vi "ConfigOperateMode.vi"(8 "error in (no error)":errorcluster, 11 "ClassIn":refnum<class "Keysight335XX.lvclass">) -> (0 "error out":errorcluster, 3 "ClassOut":refnum<class "Keysight335XX.lvclass">)   [LabVIEW 2014, in "FGenPlugins.lvlib" / "Keysight335XX.lvclass"]
uses:
  Keysight335XX.lvclass
  <instrlib>/Agilent 3352X Series/Agilent 3352X Series.lvlib
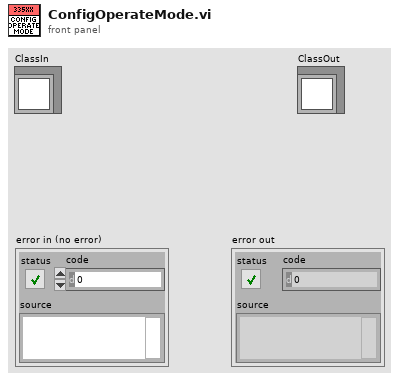
[diagram p1: front panel]
types:
  T1 = typedef "FGenPlugins.lvlib/NISTFGenPluginsBase.lvclass/ChannelParamElement.ctl" = cluster{"sName":string, "eOperateMode":u16, "bEnabled":bool, "eOutputMode":u16, "iIndex":i32, "iNameBufferSize":i32, "fGain":dbl}
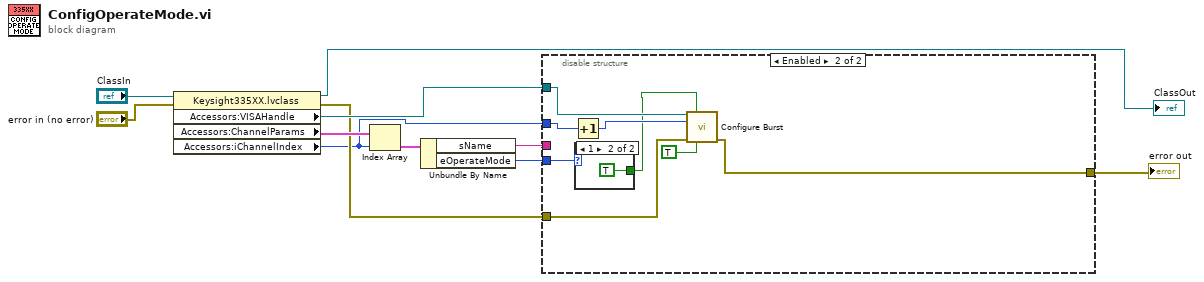
[diagram p0: block diagram]
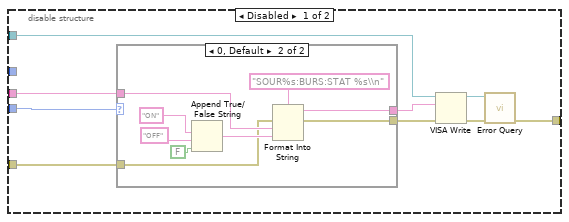
[diagram p2: hidden frame]
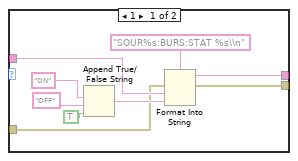
[diagram p3: hidden frame]
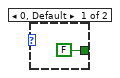
[diagram p4: hidden frame]
diagram:
  n1 = property class="Keysight335XX.lvclass"(reference="ClassIn", error in="error in (no error)") -> (reference out=→"ClassOut":refnum<class "Keysight335XX.lvclass">, error out=w6:errorcluster, "Accessors:VISAHandle"=w10:refnum<visa-resource-name>, "Accessors:ChannelParams"=w8:T1[], "Accessors:iChannelIndex"=w2:i32)
  n2 = Index Array(array=w8, index=w2) -> (element=w5:T1)
  n3 = Unbundle By Name(w5) -> ("sName"=w4:string, "eOperateMode"=w3:u16)
  n4 = disable-structure shown="Enabled" {
    disable-tunnel: w10 -> [w20 w46]
    disable-tunnel: [w19 w39] -> w9
    disable-tunnel: w6 -> [w18 w40]
    disable-tunnel: w4 -> [w13 _]
    disable-tunnel: w3 -> [w12 w43]
    disable-tunnel: w2 -> [_ w45]
    frame Disabled {
      n5 = case shown="0, Default" w12 {
        tunnel: w13 -> [w24 w33]
        tunnel: w18 -> [w23 w32]
        tunnel: [w22 w31] -> w17
        tunnel: [w21 w30] -> w16
        frame 1 {
          n6 = Append True/False String(1:TRUE ("selector"), 2:"OFF", 3:"ON") -> (0:w25:string)  [unwired: 1 out]
          n7 = Format Into String(format string="SOUR%s:BURS:STAT %s\\n", error in=w23, w24, w25) -> (resulting string=w21:string, error out=w22:errorcluster)  [unwired: 1 in]
        }
        frame 0, Default {
          n8 = Append True/False String(1:FALSE ("selector"), 2:"OFF", 3:"ON") -> (0:w34:string)  [unwired: 1 out]
          n9 = Format Into String(format string="SOUR%s:BURS:STAT %s\\n", error in=w32, w33, w34) -> (resulting string=w30:string, error out=w31:errorcluster)  [unwired: 1 in]
        }
      }
      n10 = VISA Write(VISA resource name=w20, write buffer=w16, error in (no error)=w17) -> (VISA resource name out=w15:refnum<visa-resource-name>, error out=w14:errorcluster)  [unwired: 1 out]
      n11 = call <instrlib>:"Error Query.vi"("error in (no error)"=w14, "VISA resource name"=w15) -> ("error out"=w19:errorcluster)  [unwired: 9 out]
    }
    frame Enabled {
      n12 = Increment(x=w45) -> (x+1=w44:i32)
      n13 = case shown="1" w43 {
        tunnel: [FALSE TRUE] -> w42
        frame 0, Default {
        }
        frame 1 {
        }
      }
      n14 = call <instrlib>:"Configure Burst.vi"("VISA resource name"=w46, "Enable Burst (T: Enable)"=w42, "Channel (1: 1)"=w44, "error in (no error)"=w40, "Infinite Cycle (T: Enable)"=TRUE) -> ("error out"=w39:errorcluster)  [unwired: 9 in, 1 out]
    }
  }
  "error out" <- w9
